vi "Lift Sensor Init.vi"(1 "error in":errorcluster) -> (0 "error out":errorcluster)   [LabVIEW 2014]
uses:
  <vilib>/Rock Robotics/SystemInterfaces/DIO/FPGA_DIOChannel.ctl
  <vilib>/Rock Robotics/SystemInterfaces/Typedef/FPGA_TypedefAnalogModule.ctl
  <vilib>/Rock Robotics/SystemInterfaces/AI/FPGA_AIChannel.ctl
  <vilib>/Rock Robotics/SystemInterfaces/Typedef/FPGA_TypedefDigitalModule.ctl
  <vilib>/Rock Robotics/WPI/Switch/WPI_SwitchOpenLimit.vi
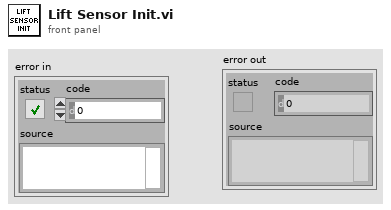
[diagram p1: front panel]
types:
  T1 = typedef "FPGA_DIOChannel.ctl" = enum8{"DIO 0", "DIO 1", "DIO 2", "DIO 3", "DIO 4", "DIO 5", "DIO 6", "DIO 7", "DIO 8", "DIO 9", "DIO MXP 0", "DIO MXP 1", "DIO MXP 2", "DIO MXP 3", "DIO MXP 4", "DIO MXP 5", "DIO MXP 6", "DIO MXP 7", "DIO MXP 8", "DIO MXP 9", "DIO MXP 10", "DIO MXP 11", "DIO MXP 12", "DIO MXP 13", "DIO MXP 14", "DIO MXP 15", "Invalid"}
  T2 = typedef "FPGA_TypedefDigitalModule.ctl" = enum16{"Controller 1"}
  T3 = typedef "FPGA_AIChannel.ctl" = enum8{"AI 0", "AI 1", "AI 2", "AI 3", "AI MXP 0", "AI MXP 1", "AI MXP 2", "AI MXP 3", "Invalid"}
  T4 = typedef "FPGA_TypedefAnalogModule.ctl" = enum16{"Controller 1"}
  T5 = typedef "WPI_SwitchDevRef.ctl" = cluster{"DevStatus":errorcluster, "DIO Channel":T1, "Controller":T2, "CntIndex":T6, "Normally Closed":bool}
  T6 = typedef "FPGA_CounterCtrSystemIndex.ctl" = enum8{"Ctr 0", "Ctr 1", "Ctr 2", "Ctr 3", "Ctr 4", "Ctr 5", "Ctr 6", "Ctr 7", "Invalid"}
  T7 = typedef "WPI_PotentiometerDevRef.ctl" = cluster{"DevStatus":errorcluster, "Controller":T4, "Analog Channel":T3, "Invert Output":bool}
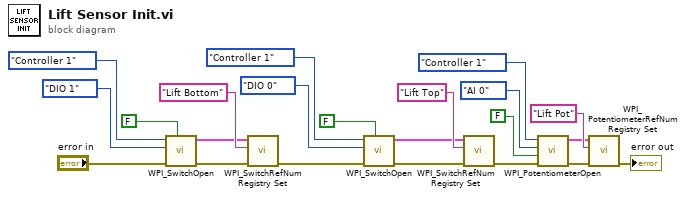
[diagram p0: block diagram]
diagram:
  n1 = call-poly <vilib>:"WPI_SwitchOpen.vi"("Normally Closed"=FALSE, "error in (no error)"="error in", "DIO Channel"=FPGA_DIOChannel."DIO 1", "Controller"=FPGA_TypedefDigitalModule."Controller 1") -> ("error out"=w21:errorcluster, "SwitchDevRef"=w20:T5)  [unwired: 6 in]
  n2 = call <vilib>:"WPI_SwitchRefNum Registry Set.vi"("error in (no error)"=w21, "refnum name"="Lift Bottom", "SwitchDevRef"=w20) -> ("error out"=w2:errorcluster)  [unwired: 7 in, 1 out]
  n3 = call-poly <vilib>:"WPI_SwitchOpen.vi"("Normally Closed"=FALSE, "error in (no error)"=w2, "DIO Channel"=FPGA_DIOChannel."DIO 0", "Controller"=FPGA_TypedefDigitalModule."Controller 1") -> ("error out"=w9:errorcluster, "SwitchDevRef"=w8:T5)  [unwired: 6 in]
  n4 = call <vilib>:"WPI_SwitchRefNum Registry Set.vi"("error in (no error)"=w9, "refnum name"="Lift Top", "SwitchDevRef"=w8) -> ("error out"=w1:errorcluster)  [unwired: 7 in, 1 out]
  n5 = call <vilib>:"WPI_PotentiometerOpen.vi"("error in (no error)"=w1, "Invert Output"=FALSE, "Analog Channel"=FPGA_AIChannel."AI 0", "Controller"=FPGA_TypedefAnalogModule."Controller 1") -> ("error out"=w16:errorcluster, "PotDevRef"=w14:T7)  [unwired: 6 in]
  n6 = call <vilib>:"WPI_PotentiometerRefNum Registry Set.vi"("error in (no error)"=w16, "refnum name"="Lift Pot", "PotDevRef"=w14) -> ("error out"=→"error out":errorcluster)  [unwired: 7 in, 1 out]
